vi "Open.vi"(4 "Max Value":dbl[](array[numeric]), 6 "Min Value":dbl[](array[numeric]), 7 "Allow multiple opens?":bool, 8 "error in (no error)":errorcluster, 10 "Channel Names":tag[](array[tag])) -> (0 "error out":errorcluster, 3 "AI Ref Out":T1)   [LabVIEW 2021, in "AI.lvlib"]
doc: "Opens a reference to one or more analog input channels. You must open a reference before you read values from an analog input channel."
uses:
  <vilib>/myRIO/Instrument Drivers/Onboard IO/AI/AI.lvlib
  <vilib>/myRIO/Instrument Drivers/Onboard IO/AI/typedefs/AI Reference.ctl
  <vilib>/myRIO/Common/Instrument Driver Framework/Utilities/typedefs/myRIO Generic Hardware Reference.ctl
  <vilib>/myRIO/Common/Instrument Driver Framework/Utilities/typedefs/Hardware Version Enum.ctl
  <vilib>/myRIO/Common/Instrument Driver Framework/Utilities/typedefs/myRIO v1.0 Reference.ctl
  <vilib>/myRIO/Common/Instrument Driver Framework/Utilities/typedefs/Generic FPGA Reference.ctl
  <vilib>/myRIO/Common/Instrument Driver Framework/myRIO v1.0/AI/typedefs/AI Channels List.ctl
  <vilib>/myRIO/Common/Instrument Driver Framework/myRIO v1.0/AI/typedefs/AI Channels Enum.ctl
  <vilib>/myRIO/Common/Instrument Driver Framework/Utilities/typedefs/Analog Scaling Constants List.ctl
  <vilib>/myRIO/Common/Instrument Driver Framework/Utilities/typedefs/Analog Scaling Constants.ctl
  <vilib>/myRIO/Common/Instrument Driver Framework/Utilities/vis/Validate Channels.vi
  <vilib>/myRIO/Common/Instrument Driver Framework/myRIO v1.0/AI/vis/myRIO v1.0 Reserve AI.vi
  <vilib>/myRIO/Common/Instrument Driver Framework/roboRIO v1.0/AI/vis/roboRIO v1.0 Reserve AI.vi
  <vilib>/myRIO/Common/Instrument Driver Framework/ELVIS III v1.0/AI/vis/ELVIS III v1.0 Reserve AI.vi
  <vilib>/myRIO/Common/Instrument Driver Framework/myRIO v1.0/AI/vis/myRIO v1.0 Build MUX Configuration AI.vi
  <vilib>/myRIO/Common/Instrument Driver Framework/myRIO v1.0/Resource Manager/vis/myRIO v1.0 Reserve Channel List.vi
  <vilib>/myRIO/Common/Instrument Driver Framework/roboRIO v1.0/Resource Manager/vis/roboRIO v1.0 Reserve Channel List.vi
  <vilib>/myRIO/Common/Instrument Driver Framework/roboRIO v1.0/AI/vis/roboRIO v1.0 Build MUX Configuration AI.vi
  <vilib>/myRIO/Common/Instrument Driver Framework/ELVIS III v1.0/AI/vis/ELVIS III v1.0 Build MUX Configuration AI.vi
  <vilib>/myRIO/Common/Instrument Driver Framework/myRIO v1.0/Resource Manager/vis/myRIO v1.0 Reserve Channel.vi
  <vilib>/myRIO/Common/Instrument Driver Framework/myRIO v1.0/Resource Manager/vis/myRIO v1.0 Unreserve Channel.vi
  <vilib>/myRIO/Common/Instrument Driver Framework/roboRIO v1.0/Resource Manager/vis/roboRIO v1.0 Reserve Channel.vi
  <vilib>/myRIO/Common/Instrument Driver Framework/roboRIO v1.0/Resource Manager/vis/roboRIO v1.0 Unreserve Channel.vi
  <vilib>/myRIO/Common/Instrument Driver Framework/myRIO v1.0/Resource Manager/vis/myRIO v1.0 Build Mutex Name.vi
  <vilib>/myRIO/Common/Instrument Driver Framework/roboRIO v1.0/Resource Manager/vis/roboRIO v1.0 Build Mutex Name.vi
  <vilib>/Utility/VariantDataType/GetNumericInfo.vi
  <vilib>/myRIO/Common/Instrument Driver Framework/myRIO v1.0/AI/vis/myRIO v1.0 Get Scaling Constants AI.vi
  <vilib>/myRIO/Common/Instrument Driver Framework/Utilities/vis/IO Manager.vi
  <vilib>/myRIO/Common/Instrument Driver Framework/Utilities/vis/Configuration Manager.vi
  <vilib>/myRIO/Common/Instrument Driver Framework/myRIO v1.0/myRIO v1.0 Close.vi
  <vilib>/myRIO/Common/Instrument Driver Framework/roboRIO v1.0/AI/vis/roboRIO v1.0 Get Scaling Constants AI.vi
  <vilib>/myRIO/Common/Instrument Driver Framework/ELVIS III v1.0/Resource Manager/vis/ELVIS III v1.0 Coerce AI Scaling.vi
  <vilib>/myRIO/Common/Instrument Driver Framework/ELVIS III v1.0/Resource Manager/vis/ELVIS III v1.0 Reserve Channel List.vi
  <vilib>/myRIO/Common/Instrument Driver Framework/ELVIS III v1.0/Resource Manager/vis/ELVIS III v1.0 Configure AI Mode.vi
  <vilib>/userdefined/High Color/nirio_resource_hc.ctl
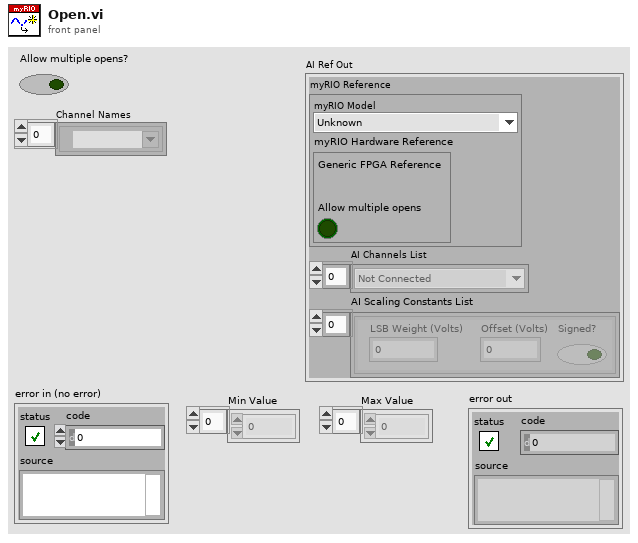
[diagram p1: front panel]
types:
  T1 = typedef "AI.lvlib/AI Reference.ctl" = cluster{"myRIO Reference":T2, "AI Channels List":T6, "AI Scaling Constants List":T8}
  T2 = typedef "myRIO Generic Hardware Reference.ctl" = cluster{"myRIO Model":T3, "myRIO Hardware Reference":T4}
  T3 = typedef "Hardware Version Enum.ctl" = enum16{"Unknown", "myRIO-1900", "myRIO-1950", "roboRIO", "NI ELVIS RIO CM", "ELVIS III"}
  T4 = typedef "myRIO v1.0 Reference.ctl" = cluster{"Generic FPGA Reference":T5, "Allow multiple opens":bool}
  T5 = typedef "Generic FPGA Reference.ctl" = refnum<k20>
  T6 = typedef "AI Channels List.ctl" = T7[]
  T7 = typedef "AI Channels Enum.ctl" = enum16{"Not Connected", "AudioIn/Left", "AudioIn/Right", "C/AI0", "C/AI1", "A/AI0", "A/AI1", "A/AI2", "A/AI3", "A/AI4", "A/AI5", "A/AI6", "A/AI7", "B/AI0", "B/AI1", "B/AI2", "B/AI3", "B/AI4", "B/AI5", "B/AI6", "B/AI7", "AI/AI0", "AI/AI1", "AI/AI2", "AI/AI3", "A/AI0 (DIFF)", "A/AI1 (DIFF)", "A/AI2 (DIFF)", "A/AI3 (DIFF)", "B/AI0 (DIFF)", "B/AI1 (DIFF)", "B/AI2 (DIFF)", "B/AI3 (DIFF)"}
  T8 = typedef "Analog Scaling Constants List.ctl" = T9[]
  T9 = typedef "Analog Scaling Constants.ctl" = cluster{"LSB Weight (Volts)":dbl, "Offset (Volts)":dbl, "Signed?":bool}
  T10 = typedef "nirio_resource_hc.ctl" = tag
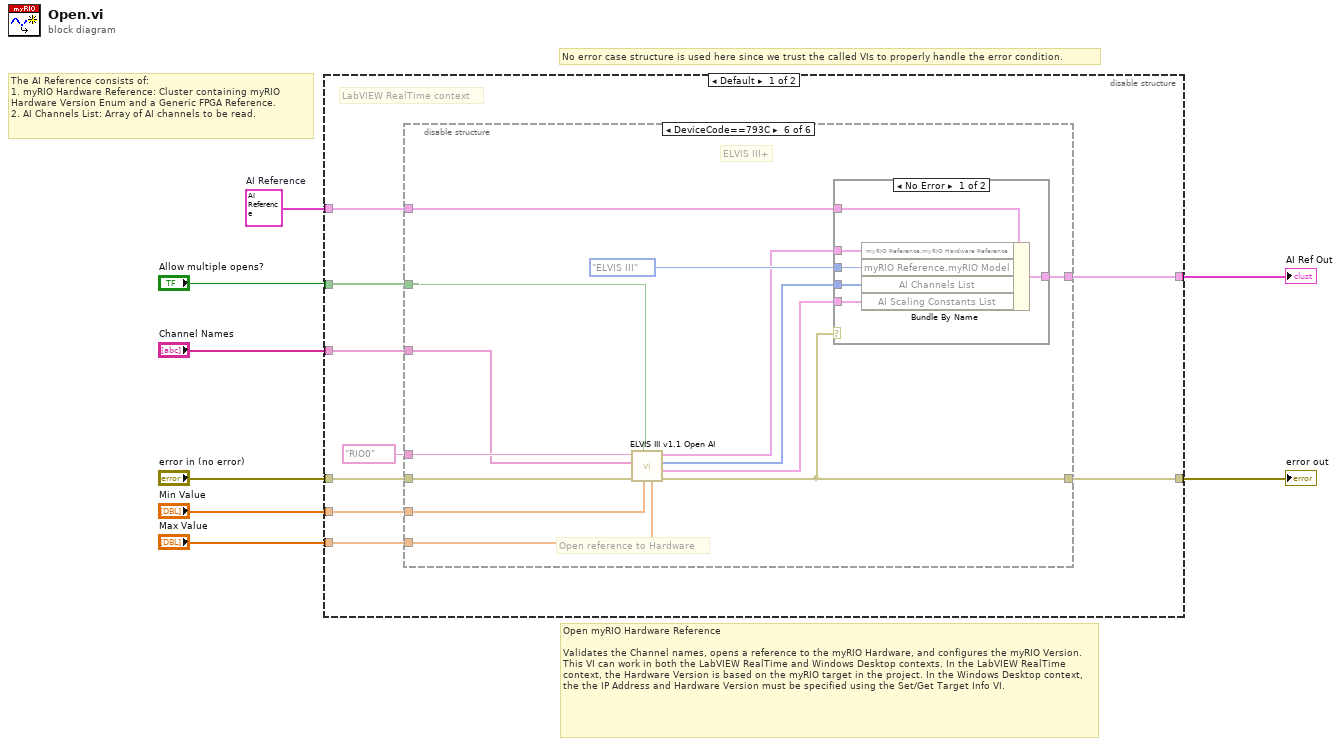
[diagram p0: block diagram]
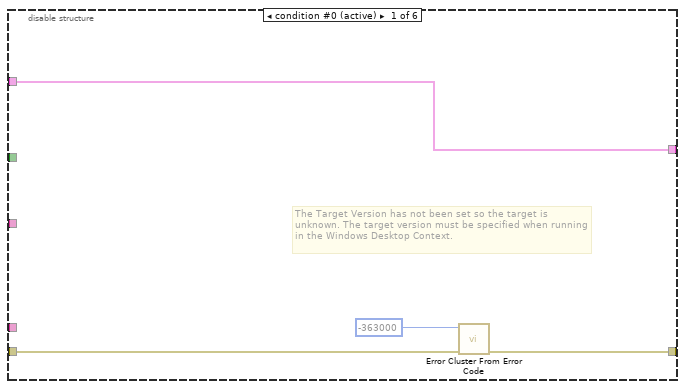
[diagram p2: hidden frame]
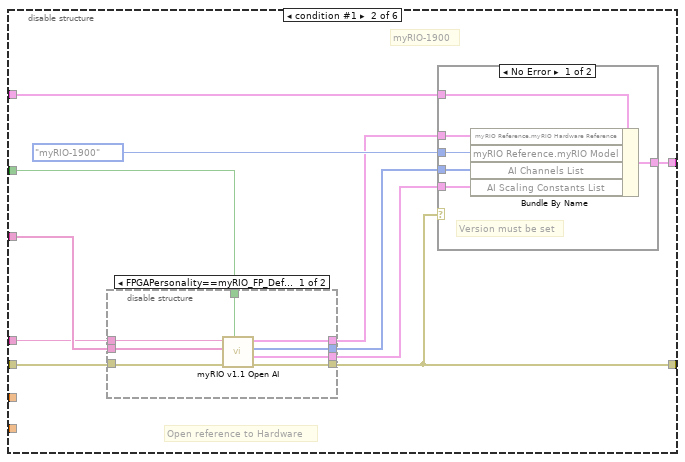
[diagram p3: hidden frame]
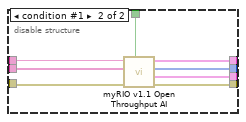
[diagram p4: hidden frame]
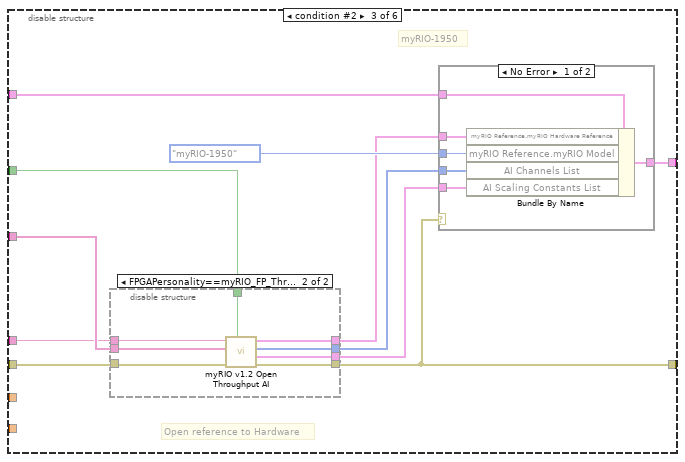
[diagram p6: hidden frame]
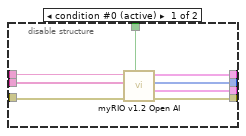
[diagram p7: hidden frame]
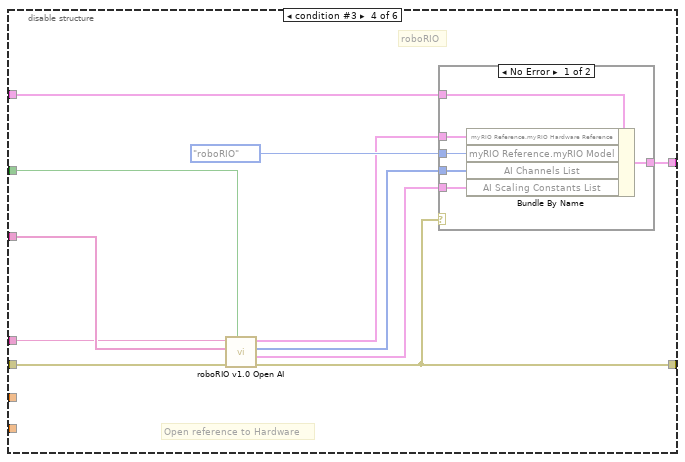
[diagram p9: hidden frame]
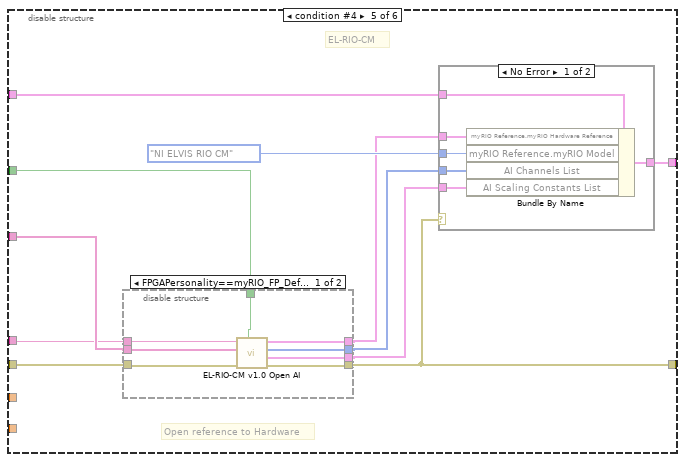
[diagram p11: hidden frame]
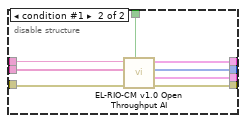
[diagram p12: hidden frame]
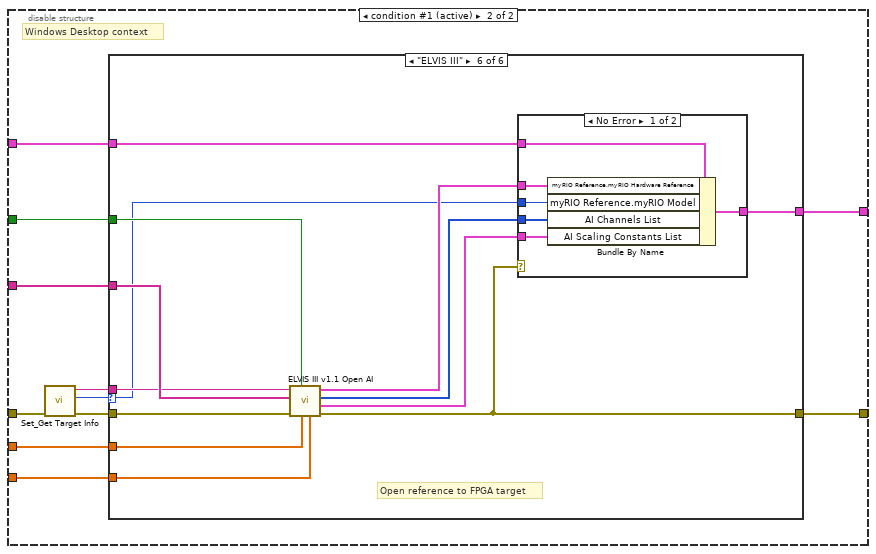
[diagram p15: hidden frame]
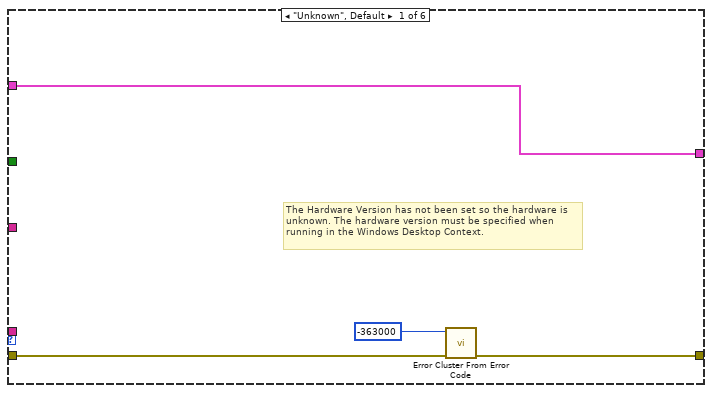
[diagram p16: hidden frame]
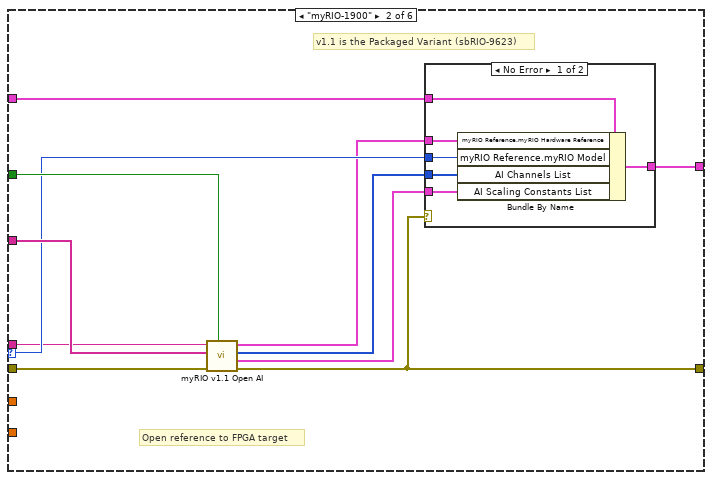
[diagram p17: hidden frame]
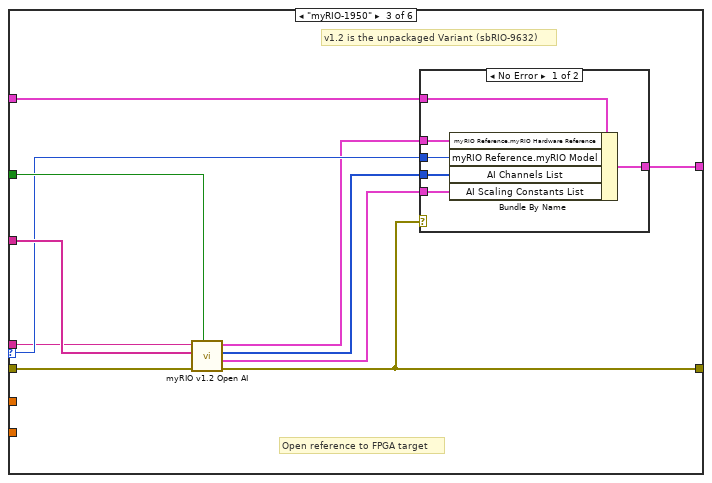
[diagram p19: hidden frame]
diagram:
  w4 = T1 {"myRIO Reference"={"myRIO Model"=enum."Unknown", "myRIO Hardware Reference"={"Generic FPGA Reference"=refnum, "Allow multiple opens"=FALSE}}, "AI Channels List"=[], "AI Scaling Constants List"=[]}  # AI Reference
  # "No error case structure is used here since we trust the called VIs to properly handle the error condition."
  # "The AI Reference consists of:\n1. myRIO Hardware Reference: Cluster containing myRIO Hardware Version Enum and a Generic FPGA Reference.\n2. AI Channels List: Array of AI channels to be read."
  # "Open myRIO Hardware Reference\n\nValidates the Channel names, opens a reference to the myRIO Hardware, and configures the myRIO Version. This VI can work in both the LabVIEW RealTime and Windows Desktop contexts. In the LabVIEW RealTime context, the Hardware Version is based on the myRIO target in the project. In the Windows Desktop context, the the IP Address and Hardware Version must be specified using the Set/Get Target Info VI."
  n1 = disable-structure shown="Default" {
    disable-tunnel: [w17 w171] -> w5
    disable-tunnel: "Channel Names" -> [w16 w168]
    disable-tunnel: "Allow multiple opens?" -> [w15 w170]
    disable-tunnel: [w14 w169] -> w3
    disable-tunnel: "error in (no error)" -> [w13 w167]
    disable-tunnel: w4 -> [w12 w166]
    disable-tunnel: "Max Value" -> [w10 w162]
    disable-tunnel: "Min Value" -> [w9 w163]
    frame condition #0 {
      # "LabVIEW RealTime context"
      n2 = disable-structure shown="DeviceCode==793C" {
        disable-tunnel: [w21 w24 w57 w91 w115 w142] -> w17
        disable-tunnel: w16 -> [_ w32 w66 w100 w110 w147]
        disable-tunnel: w15 -> [_ w28 w65 w99 w108 w149]
        disable-tunnel: [w18 w31 w64 w98 w118 w143] -> w14
        disable-tunnel: w13 -> [w20 w29 w62 w96 w111 w146]
        disable-tunnel: w12 -> [w18 w27 w60 w94 w116 w150]
        disable-tunnel: T10 "RIO0" ("Resource name") -> [_ w25 w58 w92 w109 w148]
        disable-tunnel: w10 -> [_ _ _ _ _ w144]
        disable-tunnel: w9 -> [_ _ _ _ _ w145]
        frame condition #0 (active) {
          # "The Target Version has not been set so the target is unknown. The target version must be specified when running in the Windows Desktop Context."
          n3 = call <vilib>:"Error Cluster From Error Code.vi"("error in (no error)"=w20, "error code (0)"=-363000) -> ("error out"=w21:errorcluster)  [unwired: 7 in]
        }
        frame condition #1 {
          # "myRIO-1900"
          # "Open reference to Hardware"
          n4 = disable-structure shown="FPGAPersonality==myRIO_FP_Default, Default" {
            disable-tunnel: w32 -> [w40 w48]
            disable-tunnel: w29 -> [w39 w47]
            disable-tunnel: w28 -> [w38 w46]
            disable-tunnel: [w37 w45] -> w26
            disable-tunnel: w25 -> [w36 w44]
            disable-tunnel: [w35 w43] -> w24
            disable-tunnel: [w34 w42] -> w23
            disable-tunnel: [w33 w41] -> w22
            frame condition #0 (active) {
              n5 = call <vilib>:"myRIO v1.1 Open AI.vi"("Allow multiple opens?"=w38, "error in (no error)"=w39, "Channel Names"=w40, "Resource name"=w36) -> ("error out"=w35:errorcluster, "AI Scale Constants List"=w33:T8, "AI Channel List"=w37:T6, "myRIO Ref Out"=w34:T4)  [unwired: 4 in]
            }
            frame condition #1 {
              n6 = call <vilib>:"myRIO v1.1 Open Throughput AI.vi"("Allow multiple opens?"=w46, "error in (no error)"=w47, "Channel Names"=w48, "Resource name"=w44) -> ("error out"=w43:errorcluster, "AI Scale Constants List"=w41:T8, "AI Channel List"=w45:T6, "myRIO Ref Out"=w42:T4)  [unwired: 4 in]
            }
          }
          n7 = case shown="No Error" w24 {
            tunnel: [w54 w55] -> w31
            tunnel: Hardware_Version_Enum."myRIO-1900" ("Hardware Version Enum") -> [w53 _]
            tunnel: w27 -> [w52 w55]
            tunnel: w26 -> [w51 _]
            tunnel: w23 -> [w50 _]
            tunnel: w22 -> [w49 _]
            frame No Error {
              # "Version must be set"
              n8 = Bundle By Name(cluster=w52, "myRIO Reference.myRIO Hardware Reference"=w50, "myRIO Reference.myRIO Model"=w53, "AI Channels List"=w51, "AI Scaling Constants List"=w49) -> (w54:T1)
            }
            frame Error {
            }
          }
        }
        frame condition #2 {
          # "myRIO-1950"
          # "Open reference to Hardware"
          n9 = disable-structure shown="FPGAPersonality==myRIO_FP_Throughput" {
            disable-tunnel: w66 -> [w74 w82]
            disable-tunnel: w65 -> [w73 w81]
            disable-tunnel: w62 -> [w72 w80]
            disable-tunnel: [w71 w79] -> w61
            disable-tunnel: [w70 w78] -> w59
            disable-tunnel: w58 -> [w69 w77]
            disable-tunnel: [w68 w76] -> w57
            disable-tunnel: [w67 w75] -> w56
            frame condition #0 (active) {
              n10 = call <vilib>:"myRIO v1.2 Open AI.vi"("Allow multiple opens?"=w73, "error in (no error)"=w72, "Channel Names"=w74, "Resource name"=w69) -> ("error out"=w68:errorcluster, "AI Scale Constants List"=w67:T8, "AI Channel List"=w70:T6, "myRIO Ref Out"=w71:T4)  [unwired: 4 in]
            }
            frame condition #1 {
              n11 = call <vilib>:"myRIO v1.2 Open Throughput AI.vi"("Allow multiple opens?"=w81, "error in (no error)"=w80, "Channel Names"=w82, "Resource name"=w77) -> ("error out"=w76:errorcluster, "AI Scale Constants List"=w75:T8, "AI Channel List"=w78:T6, "myRIO Ref Out"=w79:T4)  [unwired: 4 in]
            }
          }
          n12 = case shown="No Error" w57 {
            tunnel: [w88 w89] -> w64
            tunnel: Hardware_Version_Enum."myRIO-1950" ("Hardware Version Enum") -> [w87 _]
            tunnel: w61 -> [w84 _]
            tunnel: w60 -> [w86 w89]
            tunnel: w59 -> [w85 _]
            tunnel: w56 -> [w83 _]
            frame No Error {
              n13 = Bundle By Name(cluster=w86, "myRIO Reference.myRIO Hardware Reference"=w84, "myRIO Reference.myRIO Model"=w87, "AI Channels List"=w85, "AI Scaling Constants List"=w83) -> (w88:T1)
            }
            frame Error {
            }
          }
        }
        frame condition #3 {
          # "roboRIO"
          # "Open reference to Hardware"
          n14 = call <vilib>:"roboRIO v1.0 Open AI.vi"("Allow multiple opens?"=w99, "error in (no error)"=w96, "Channel Names"=w100, "Resource name"=w92) -> ("error out"=w91:errorcluster, "AI Scale Constants List"=w90:T8, "AI Channel List"=w93:T6, "myRIO Ref Out"=w95:T4)  [unwired: 4 in]
          n15 = case shown="No Error" w91 {
            tunnel: [w106 w107] -> w98
            tunnel: Hardware_Version_Enum."roboRIO" ("Hardware Version Enum") -> [w105 _]
            tunnel: w95 -> [w102 _]
            tunnel: w94 -> [w104 w107]
            tunnel: w93 -> [w103 _]
            tunnel: w90 -> [w101 _]
            frame No Error {
              n16 = Bundle By Name(cluster=w104, "myRIO Reference.myRIO Hardware Reference"=w102, "myRIO Reference.myRIO Model"=w105, "AI Channels List"=w103, "AI Scaling Constants List"=w101) -> (w106:T1)
            }
            frame Error {
            }
          }
        }
        frame condition #4 {
          # "EL-RIO-CM"
          # "Open reference to Hardware"
          n17 = disable-structure shown="FPGAPersonality==myRIO_FP_Default, Default" {
            disable-tunnel: w110 -> [w121 w134]
            disable-tunnel: w108 -> [w119 w133]
            disable-tunnel: w111 -> [w120 w132]
            disable-tunnel: [w123 w131] -> w112
            disable-tunnel: [w124 w130] -> w113
            disable-tunnel: w109 -> [w122 w129]
            disable-tunnel: [w126 w128] -> w115
            disable-tunnel: [w125 w127] -> w114
            frame condition #0 (active) {
              n18 = call <vilib>:"EL-RIO-CM v1.0 Open AI.vi"("Allow multiple opens?"=w119, "error in (no error)"=w120, "Channel Names"=w121, "Resource name"=w122) -> ("error out"=w126:errorcluster, "AI Scale Constants List"=w125:T8, "AI Channel List"=w124:T6, "myRIO Ref Out"=w123:T4)  [unwired: 4 in]
            }
            frame condition #1 {
              n19 = call <vilib>:"EL-RIO-CM v1.0 Open Throughput AI.vi"("Allow multiple opens?"=w133, "error in (no error)"=w132, "Channel Names"=w134, "Resource name"=w129) -> ("error out"=w128:errorcluster, "AI Scale Constants List"=w127:T8, "AI Channel List"=w130:T6, "myRIO Ref Out"=w131:T4)  [unwired: 4 in]
            }
          }
          n20 = case shown="No Error" w115 {
            tunnel: [w140 w141] -> w118
            tunnel: Hardware_Version_Enum."NI ELVIS RIO CM" ("Hardware Version Enum") -> [w139 _]
            tunnel: w112 -> [w136 _]
            tunnel: w116 -> [w138 w141]
            tunnel: w113 -> [w137 _]
            tunnel: w114 -> [w135 _]
            frame No Error {
              n21 = Bundle By Name(cluster=w138, "myRIO Reference.myRIO Hardware Reference"=w136, "myRIO Reference.myRIO Model"=w139, "AI Channels List"=w137, "AI Scaling Constants List"=w135) -> (w140:T1)
            }
            frame Error {
            }
          }
        }
        frame condition #5 {
          # "ELVIS III+"
          # "Open reference to Hardware"
          n22 = call <vilib>:"ELVIS III v1.1 Open AI.vi"("Max Value"=w144, "Min Value"=w145, "Allow multiple opens?"=w149, "error in (no error)"=w146, "Channel Names"=w147, "Resource name"=w148) -> ("error out"=w142:errorcluster, "AI Scale Constants List"=w153:T8, "AI Channel List"=w152:T6, "myRIO Ref Out"=w151:T4)  [unwired: 2 in]
          n23 = case shown="No Error" w142 {
            tunnel: [w160 w161] -> w143
            tunnel: Hardware_Version_Enum."ELVIS III" ("Hardware Version Enum") -> [w159 _]
            tunnel: w151 -> [w156 _]
            tunnel: w150 -> [w158 w161]
            tunnel: w152 -> [w157 _]
            tunnel: w153 -> [w155 _]
            frame No Error {
              n24 = Bundle By Name(cluster=w158, "myRIO Reference.myRIO Hardware Reference"=w156, "myRIO Reference.myRIO Model"=w159, "AI Channels List"=w157, "AI Scaling Constants List"=w155) -> (w160:T1)
            }
            frame Error {
            }
          }
        }
      }
    }
    frame condition #1 (active) {
      # "Windows Desktop context"
      n25 = call <vilib>:"Set_Get Target Info.vi"() -> ("Hardware Version"=w164:T3, "IP Address"=w165:string)  [unwired: 9 in, 1 out]
      n26 = case shown="\"ELVIS III\"" w164 {
        selector: w164 -> [_ w183 w202 w220 w238 w251]
        tunnel: [w175 w178 w196 w214 w232 w256] -> w171
        tunnel: w168 -> [_ w186 w204 w222 w240 w253]
        tunnel: w170 -> [_ w185 w203 w221 w239 w254]
        tunnel: [w172 w184 w198 w216 w234 w257] -> w169
        tunnel: w167 -> [w173 w180 w201 w219 w237 w250]
        tunnel: w165 -> [_ w182 w200 w218 w236 w252]
        tunnel: w166 -> [w172 w181 w199 w217 w235 w255]
        tunnel: w163 -> [_ _ _ _ _ w249]
        tunnel: w162 -> [_ _ _ _ _ w248]
        frame "Unknown", Default {
          # "The Hardware Version has not been set so the hardware is unknown. The hardware version must be specified when running in the Windows Desktop Context."
          n27 = call <vilib>:"Error Cluster From Error Code.vi"("error in (no error)"=w173, "error code (0)"=-363000) -> ("error out"=w175:errorcluster)  [unwired: 7 in]
        }
        frame "myRIO-1900" {
          # "v1.1 is the Packaged Variant (sbRIO-9623)"
          # "Open reference to FPGA target"
          n28 = call <vilib>:"myRIO v1.1 Open AI.vi"("Allow multiple opens?"=w185, "error in (no error)"=w180, "Channel Names"=w186, "Resource name"=w182) -> ("error out"=w178:errorcluster, "AI Scale Constants List"=w176:T8, "AI Channel List"=w179:T6, "myRIO Ref Out"=w177:T4)  [unwired: 4 in]
          n29 = case shown="No Error" w178 {
            tunnel: [w192 w193] -> w184
            tunnel: w183 -> [w191 _]
            tunnel: w181 -> [w190 w193]
            tunnel: w179 -> [w189 _]
            tunnel: w177 -> [w188 _]
            tunnel: w176 -> [w187 _]
            frame No Error {
              n30 = Bundle By Name(cluster=w190, "myRIO Reference.myRIO Hardware Reference"=w188, "myRIO Reference.myRIO Model"=w191, "AI Channels List"=w189, "AI Scaling Constants List"=w187) -> (w192:T1)
            }
            frame Error {
            }
          }
        }
        frame "myRIO-1950" {
          # "v1.2 is the unpackaged Variant (sbRIO-9632)"
          # "Open reference to FPGA target"
          n31 = call <vilib>:"myRIO v1.2 Open AI.vi"("Allow multiple opens?"=w203, "error in (no error)"=w201, "Channel Names"=w204, "Resource name"=w200) -> ("error out"=w196:errorcluster, "AI Scale Constants List"=w194:T8, "AI Channel List"=w197:T6, "myRIO Ref Out"=w195:T4)  [unwired: 4 in]
          n32 = case shown="No Error" w196 {
            tunnel: w202 -> [w210 _]
            tunnel: w199 -> [w209 w211]
            tunnel: [w208 w211] -> w198
            tunnel: w197 -> [w207 _]
            tunnel: w195 -> [w206 _]
            tunnel: w194 -> [w205 _]
            frame No Error {
              n33 = Bundle By Name(cluster=w209, "myRIO Reference.myRIO Hardware Reference"=w206, "myRIO Reference.myRIO Model"=w210, "AI Channels List"=w207, "AI Scaling Constants List"=w205) -> (w208:T1)
            }
            frame Error {
            }
          }
        }
        frame "roboRIO" {
          # "Open reference to FPGA target"
          n34 = call <vilib>:"roboRIO v1.0 Open AI.vi"("Allow multiple opens?"=w221, "error in (no error)"=w219, "Channel Names"=w222, "Resource name"=w218) -> ("error out"=w214:errorcluster, "AI Scale Constants List"=w212:T8, "AI Channel List"=w215:T6, "myRIO Ref Out"=w213:T4)  [unwired: 4 in]
          n35 = case shown="No Error" w214 {
            tunnel: w220 -> [w228 _]
            tunnel: w217 -> [w227 w229]
            tunnel: [w226 w229] -> w216
            tunnel: w215 -> [w225 _]
            tunnel: w213 -> [w224 _]
            tunnel: w212 -> [w223 _]
            frame No Error {
              n36 = Bundle By Name(cluster=w227, "myRIO Reference.myRIO Hardware Reference"=w224, "myRIO Reference.myRIO Model"=w228, "AI Channels List"=w225, "AI Scaling Constants List"=w223) -> (w226:T1)
            }
            frame Error {
            }
          }
        }
        frame "NI ELVIS RIO CM" {
          # "Open reference to FPGA target"
          n37 = call <vilib>:"EL-RIO-CM v1.0 Open AI.vi"("Allow multiple opens?"=w239, "error in (no error)"=w237, "Channel Names"=w240, "Resource name"=w236) -> ("error out"=w232:errorcluster, "AI Scale Constants List"=w230:T8, "AI Channel List"=w233:T6, "myRIO Ref Out"=w231:T4)  [unwired: 4 in]
          n38 = case shown="No Error" w232 {
            tunnel: w238 -> [w246 _]
            tunnel: w235 -> [w245 w247]
            tunnel: [w244 w247] -> w234
            tunnel: w233 -> [w243 _]
            tunnel: w231 -> [w242 _]
            tunnel: w230 -> [w241 _]
            frame No Error {
              n39 = Bundle By Name(cluster=w245, "myRIO Reference.myRIO Hardware Reference"=w242, "myRIO Reference.myRIO Model"=w246, "AI Channels List"=w243, "AI Scaling Constants List"=w241) -> (w244:T1)
            }
            frame Error {
            }
          }
        }
        frame "ELVIS III" {
          # "Open reference to FPGA target"
          n40 = call <vilib>:"ELVIS III v1.1 Open AI.vi"("Max Value"=w248, "Min Value"=w249, "Allow multiple opens?"=w254, "error in (no error)"=w250, "Channel Names"=w253, "Resource name"=w252) -> ("error out"=w256:errorcluster, "AI Scale Constants List"=w258:T8, "AI Channel List"=w260:T6, "myRIO Ref Out"=w259:T4)  [unwired: 2 in]
          n41 = case shown="No Error" w256 {
            tunnel: w251 -> [w266 _]
            tunnel: w255 -> [w265 w267]
            tunnel: [w264 w267] -> w257
            tunnel: w260 -> [w263 _]
            tunnel: w259 -> [w262 _]
            tunnel: w258 -> [w261 _]
            frame No Error {
              n42 = Bundle By Name(cluster=w265, "myRIO Reference.myRIO Hardware Reference"=w262, "myRIO Reference.myRIO Model"=w266, "AI Channels List"=w263, "AI Scaling Constants List"=w261) -> (w264:T1)
            }
            frame Error {
            }
          }
        }
      }
    }
  }
  "AI Ref Out" <- w3
  "error out" <- w5
